vi "tcp_client_lifter.vi"(8 "error in":errorcluster, 9 "port":u16=10390, 10 "addr":string="192.168.24.17", 11 "conn_id_in":refnum<k5>) -> (0 "error out":errorcluster, 1 "status":bool, 2 "Spill ID":i32, 3 "conn_id_out":refnum<k5>)   [LabVIEW 2019]
panel:
  out "Time EOS":dbl format="%#.6f"
  out "Raw data array":string[](array[string])
  out "BOS Time":dbl format="%#.6f"
  in  "stop":bool
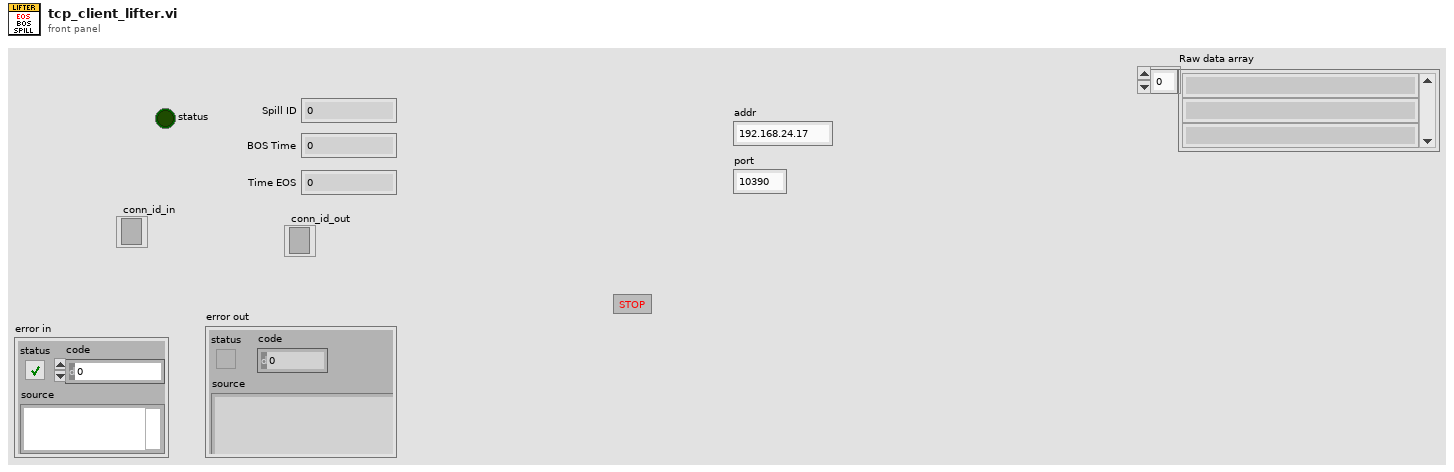
[diagram p1: front panel]
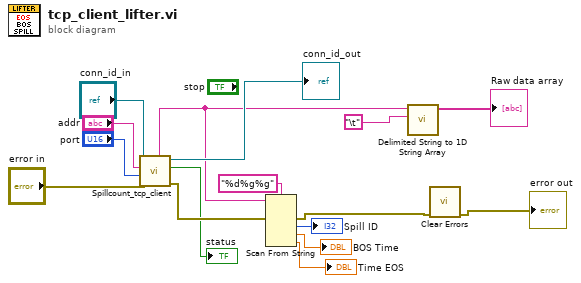
[diagram p0: block diagram]
diagram:
  n1 = call "Spillcount_tcp_client.vi"("error in"="error in", "port"="port", "address"="addr", "conn_id_in"="conn_id_in") -> ("error out"=w14:errorcluster, "status"=→"status":bool, "conn_id_out"=→"conn_id_out":refnum<k5>, "data out"=w4:string)  [unwired: 3 in, 1 out]
  n2 = Scan From String(format string="%d%g%g", input string=w4, error in=w14) -> (error out=w2:errorcluster, output 1=→"Spill ID":i32, output 2=→"BOS Time":dbl, output 3=→"Time EOS":dbl)  [unwired: 4 in, 2 out]
  n3 = call <vilib>:"Delimited String to 1D String Array.vi"("delimiter"="\t", "delimited string"=w4) -> ("string array"=→"Raw data array":string[])  [unwired: 9 in]
  n4 = call <vilib>:"Clear Errors.vi"("error in (no error)"=w2) -> ("error out"=→"error out":errorcluster)  [unwired: 5 in, 1 out]
